vi "computer name.vi"() -> (3 "name":string)   [LabVIEW 2018]
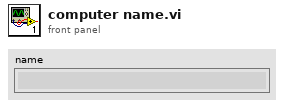
[diagram p1: front panel]
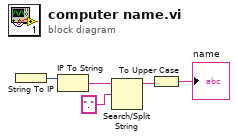
[diagram p0: block diagram]
diagram:
  n1 = String To IP() -> (0:w5:u32)  [unwired: 1 in]
  n2 = IP To String(2:w5) -> (0:w4:string)  [unwired: 1 in]
  n3 = Search/Split String(string=w4, search string/char (-)=".") -> (substring before match=w2:string)  [unwired: 1 in, 2 out]
  n4 = To Upper Case(1:w2) -> (0:→"name":string)
